vi "Tensione vapore.vi"(11 "T":dbl) -> (3 "Pv":dbl)   [LabVIEW 2019]
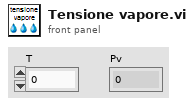
[diagram p1: front panel]
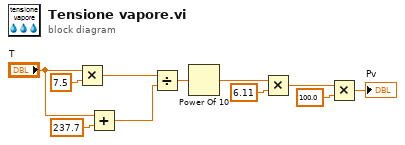
[diagram p0: block diagram]
diagram:
  n1 = Multiply(x="T", y=7.5) -> (x*y=w6:dbl)
  n2 = Add(x="T", y=237.7) -> (x+y=w9:dbl)
  n3 = Divide(x=w6, y=w9) -> (x/y=w10:dbl)
  n4 = Power Of 10(x=w10) -> (10^x=w11:dbl)
  n5 = Multiply(x=w11, y=6.11) -> (x*y=w3:dbl)
  n6 = Multiply(x=w3, y=100.0) -> (x*y=→"Pv":dbl)
